vi "Origine.vi"(0 "reference":refnum<visa-resource-name>) -> (4 "reference dup":refnum<visa-resource-name>, 8 "OK Done":bool, 15 "error out":errorcluster)   [LabVIEW 2011]
panel:
  # "Port Number 0=COM1"
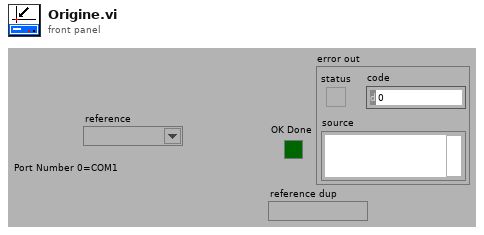
[diagram p1: front panel]
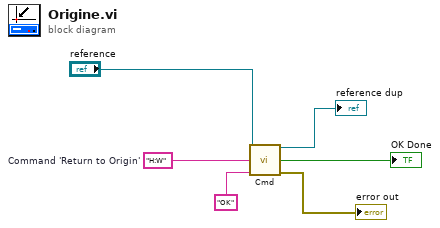
[diagram p0: block diagram]
diagram:
  w4 = "H:W"  # Command 'Return to Origin'
  n1 = call "Cmd.vi"("reference"="reference", "Command String"=w4, "String to receive"="OK") -> ("reference dup"=→"reference dup":refnum<visa-resource-name>, "OK Done"=→"OK Done":bool, "error out"=→"error out":errorcluster)  [unwired: 10 in]
